vi "Connected.vi"(8 "error in (no error)":errorcluster, 9 "Message Stream":refnum<class "Message Stream.lvclass">, 10 "Endpoint Enqueuer":refnum<class "Message Enqueuer.lvclass">, 11 "Client in":refnum<class "Client.lvclass">) -> (0 "error out":errorcluster, 3 "Client out":refnum<class "Client.lvclass">)   [LabVIEW 2021, in "Client.lvlib" / "Client.lvclass"]
uses:
  Client.lvclass
  <vilib>/ActorFramework/Message Enqueuer/Message Enqueuer.lvclass
  <vilib>/NI/Actors/Network Endpoint Actors/Abstract Classes/Message Stream/Message Stream.lvclass
  Client.lvclass/Client.ctl
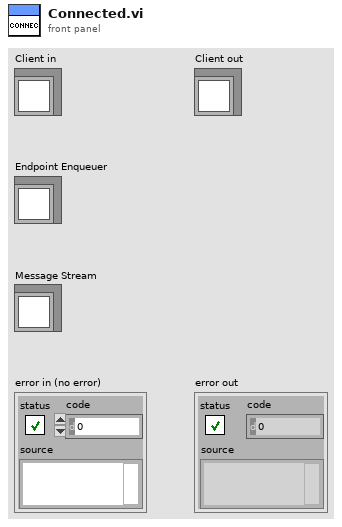
[diagram p1: front panel]
types:
  T1 = enum8{"Enabled", "Disabled", "Disabled and Grayed Out"}
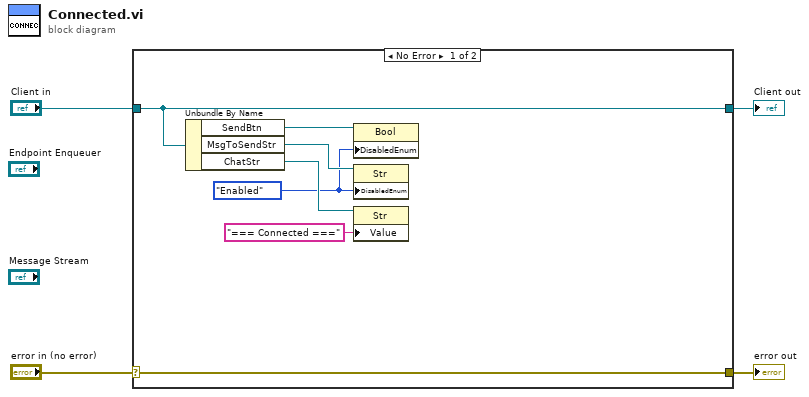
[diagram p0: block diagram]
diagram:
  n1 = case shown="No Error" "error in (no error)" {
    selector: "error in (no error)" -> [w11 w13]
    tunnel: [w11 w13] -> w3
    tunnel: [w5 w12] -> w1
    tunnel: "Client in" -> [w5 w12]
    frame No Error {
      w7 = T1."Enabled" ("Disabled")
      n2 = Unbundle By Name(w5) -> ("SendBtn"=w10:refnum<vi>, "MsgToSendStr"=w9:refnum<vi>, "ChatStr"=w8:refnum<vi>)
      n3 = property class="Bool"(reference=w10, "DisabledEnum"=w7) -> ()  [unwired: 1 in, 2 out]
      n4 = property class="Str"(reference=w9, "DisabledEnum"=w7) -> ()  [unwired: 1 in, 2 out]
      n5 = property class="Str"(reference=w8, "Value"="=== Connected ===") -> ()  [unwired: 1 in, 2 out]
    }
    frame Error {
    }
  }
  "error out" <- w3
  "Client out" <- w1
